vi "ReRemplissageGraphique.vi"(9 "XY graph ref":refnum<vi>, 10 "Y arr ref":refnum<vi>, 11 "X arr ref":refnum<vi>) -> ()   [LabVIEW 2013]
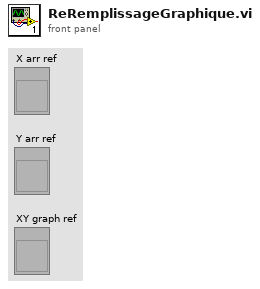
[diagram p1: front panel]
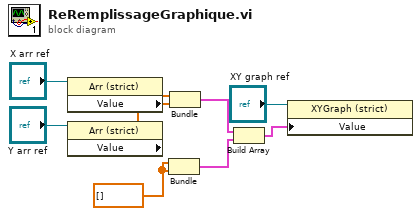
[diagram p0: block diagram]
diagram:
  w6 = dbl[] []
  n1 = property class="Arr (strict)"(reference="X arr ref") -> ("Value"=w4:dbl[])  [unwired: 1 in, 2 out]
  n2 = property class="Arr (strict)"(reference="Y arr ref") -> ("Value"=w5:dbl[])  [unwired: 1 in, 2 out]
  n3 = Bundle(w6, w6) -> (w8:cluster{dbl[], dbl[]})  [unwired: 1 in]
  n4 = Bundle("Value"=w4, "Value"=w5) -> (w7:cluster{"Value":dbl[], "Value":dbl[]})  [unwired: 1 in]
  n5 = Build Array(w7, w8) -> (w9:cluster{"Value":dbl[], "Value":dbl[]}[])
  n6 = property class="XYGraph (strict)"(reference="XY graph ref", "Value"=w9) -> ()  [unwired: 1 in, 2 out]
